vi "3_Axis_magmeter_MAIN.vi"() -> ()   [LabVIEW 2013]
doc: "Программа для обработки и визуализации трех компонент магнитного поля прибора, разработаного инженерами НЭОиКН ЛФВЭ ОИЯИ 2014"
uses:
  Magmeter.ctl
  <vilib>/Instr/_visa.llb/VISA Configure Serial Port (Instr).vi
panel:
  out "Dx Sum":u64
  in  "Порт":refnum<visa-resource-name>="COM4"
  out "Соединение":bool
  out "Err msg":string=" INSTRUCTIONS:\r\rNormal Use:  When using subVIs that incorporate the error in/error out (or error I/O) structure, place this handler where you want to inform the user of an error, typically at the end of the I/O data path, as the last action of the program.  If the error in error? is ERROR, the handler creates a message describing the error and its source.  If the type of dialog = 1 (default), the message is displayed to the user, who can only acknowedge it.  If the type = 2, the user can acknowledge the message or abort execution; aborting a program with active I/O is not recommended.  If the type = 0, no message is displayed; this is used to process the error programmatically, and the error out cluster elements are wired to individual terminals for that reason.  \r\rOther Use:\n\r\nlocal testing.  To test the error code of a subVI or function that does not have the error I/O structure, you can wire its error code and a source string to the local error code and error source inputs.  If error in error? indicates no error and error code is not equal to 0, the local code and source are substituted for the error in values, and error? is set TRUE (ERROR)."
  in  "Бод.":u32=9600
  out "i":i32
  in  "number of data sample":u64
  in  "Автосохранение":bool
  in  "Интервал \n\n[сек.]":u32=10 min=1 max=30000 step=1
  in  "Маркеры":bool
  out "Table num index":u32
  in  "Удалить измерение":bool
  in  "RXd number":u64
  in  "Dz, мм":u64=5 min=1
  in  "зафиксировать измерение":bool
  in  "Измерений\n \nна графике":u16=100
  in  "Очистить историю":bool
  in  "H макс":dbl=8.0 format="%#.1f"
  in  "H мин":dbl=-8.0 format="%#.1f"
  in  "Уст. ноль":bool
  in  "Сохранен!":bool
  in  "Plot.Visible Z":bool
  out "By":dbl format="%.3f"
  out "Bz":dbl format="%.3f"
  in  "Plot.Visible X":bool
  out "Bx":dbl format="%.3f"
  in  "Plot.Visible Y":bool
  in  "Графики толще":bool=TRUE
  in  "Стоп":bool
  out "Магнитные измерения":T1(graph)
  in  "Measurment Fl":bool
  out "Сохраненные измерения":string[][](table)
  out "Путь к файлу":path
  # "Гаусс"
  # "Результаты\nизмерений"
  # "ГС"
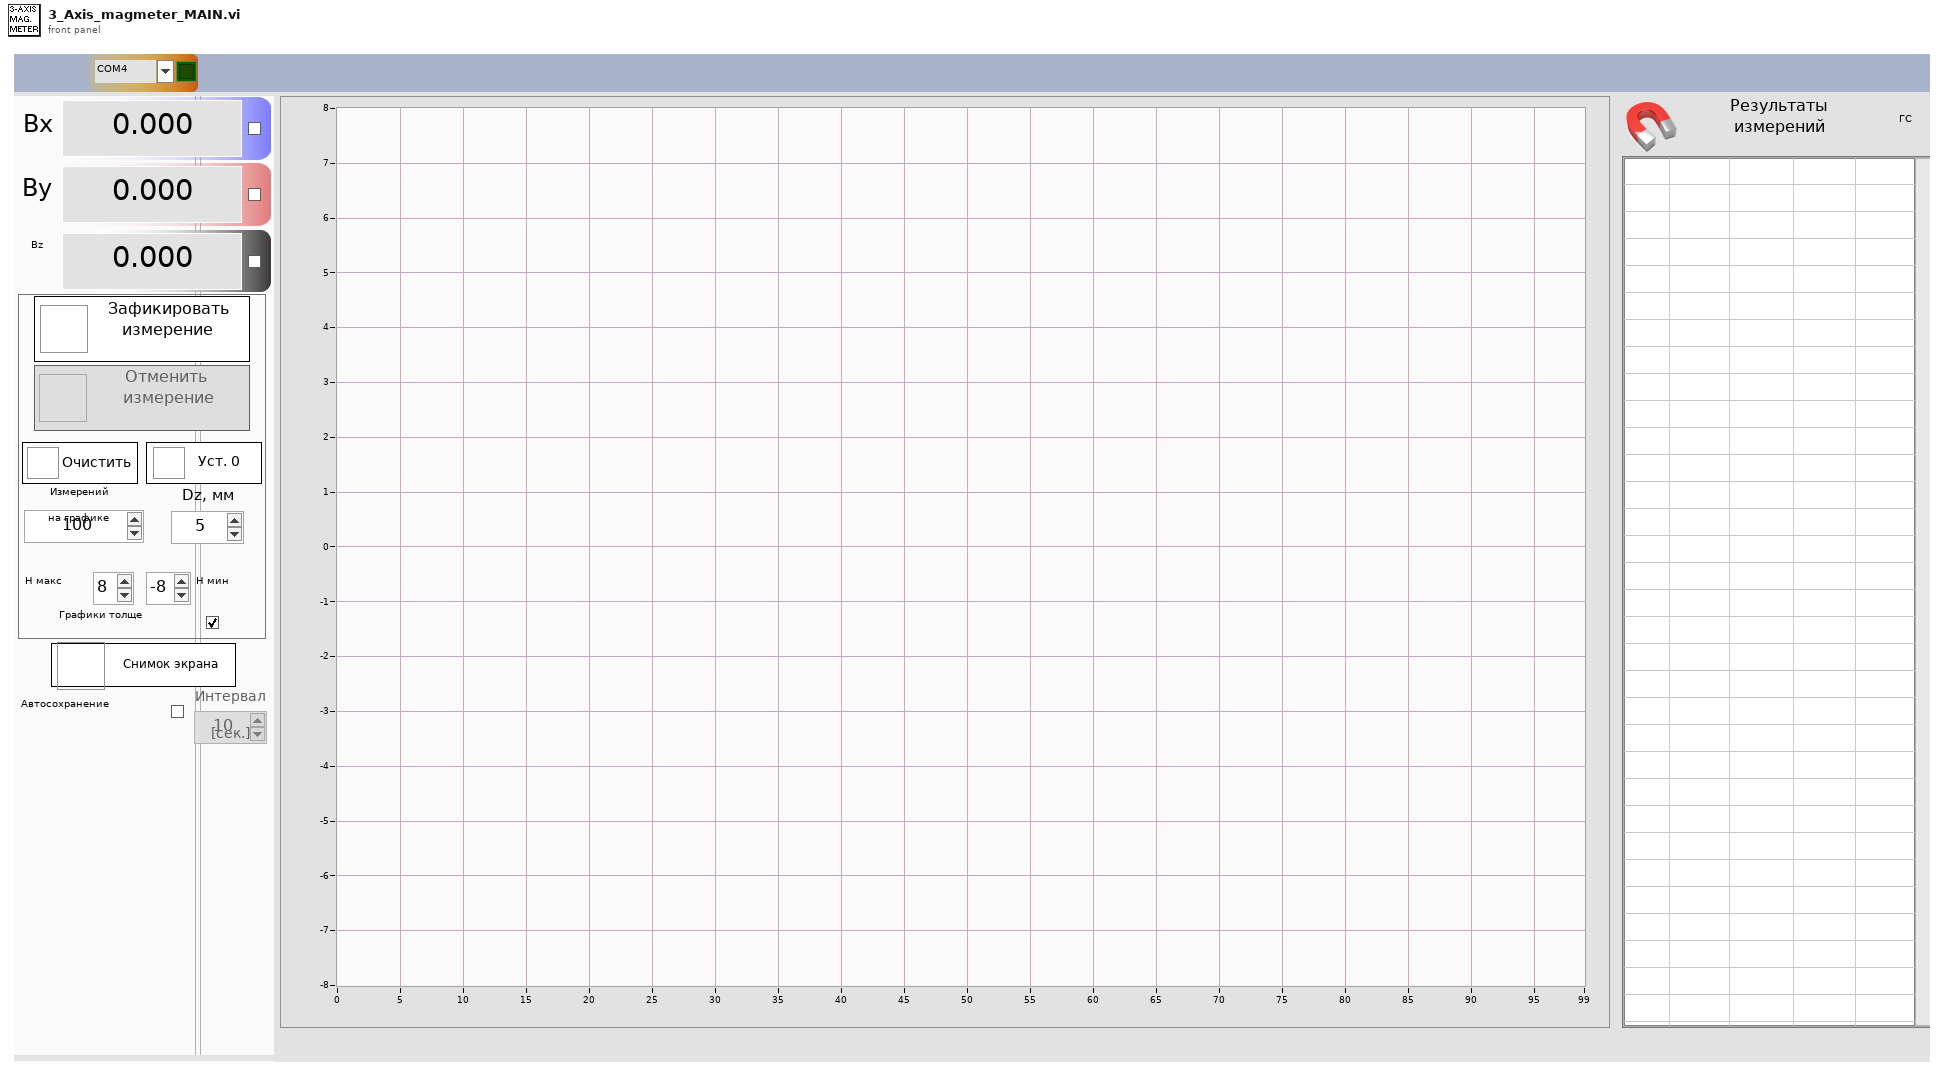
[diagram p1: front panel]
types:
  T1 = cluster{"X":dbl, "Y":dbl, "Z":dbl, "Active Plot":dbl}[]
  T2 = typedef "Magmeter.ctl" = enum16{"Initialize", "Read port", "Write port", "Stop"}
  T3 = cluster{"Value":dbl, "Value":dbl, "Value":dbl, "Active Plot":dbl}
  T4 = cluster{"Value":dbl, "Value":dbl, "Value":dbl, "X":dbl}
  T5 = cluster{"Value":dbl, "Value":dbl, "Value":dbl, "X":dbl}[]
  T6 = typedef "imagedata.ctl" = cluster{"image type":i32, "image depth":i32, "image":u8[], "mask":u8[], "colors":u32[], "Rectangle":cluster{"left":i16, "top":i16, "right":i16, "bottom":i16}}
  T7 = cluster{"read buffer":string, "serial out":refnum<visa-resource-name>, "error out":errorcluster, "occurrence":refnum<k4>}
  T8 = cluster{"out string":string, "Visa name out":refnum<visa-resource-name>, "error out":errorcluster, "occurrence":refnum<k4>}
  T9 = cluster{"Visa name out":refnum<visa-resource-name>, "error out":errorcluster, "status":bool, "occurrence":refnum<k4>}
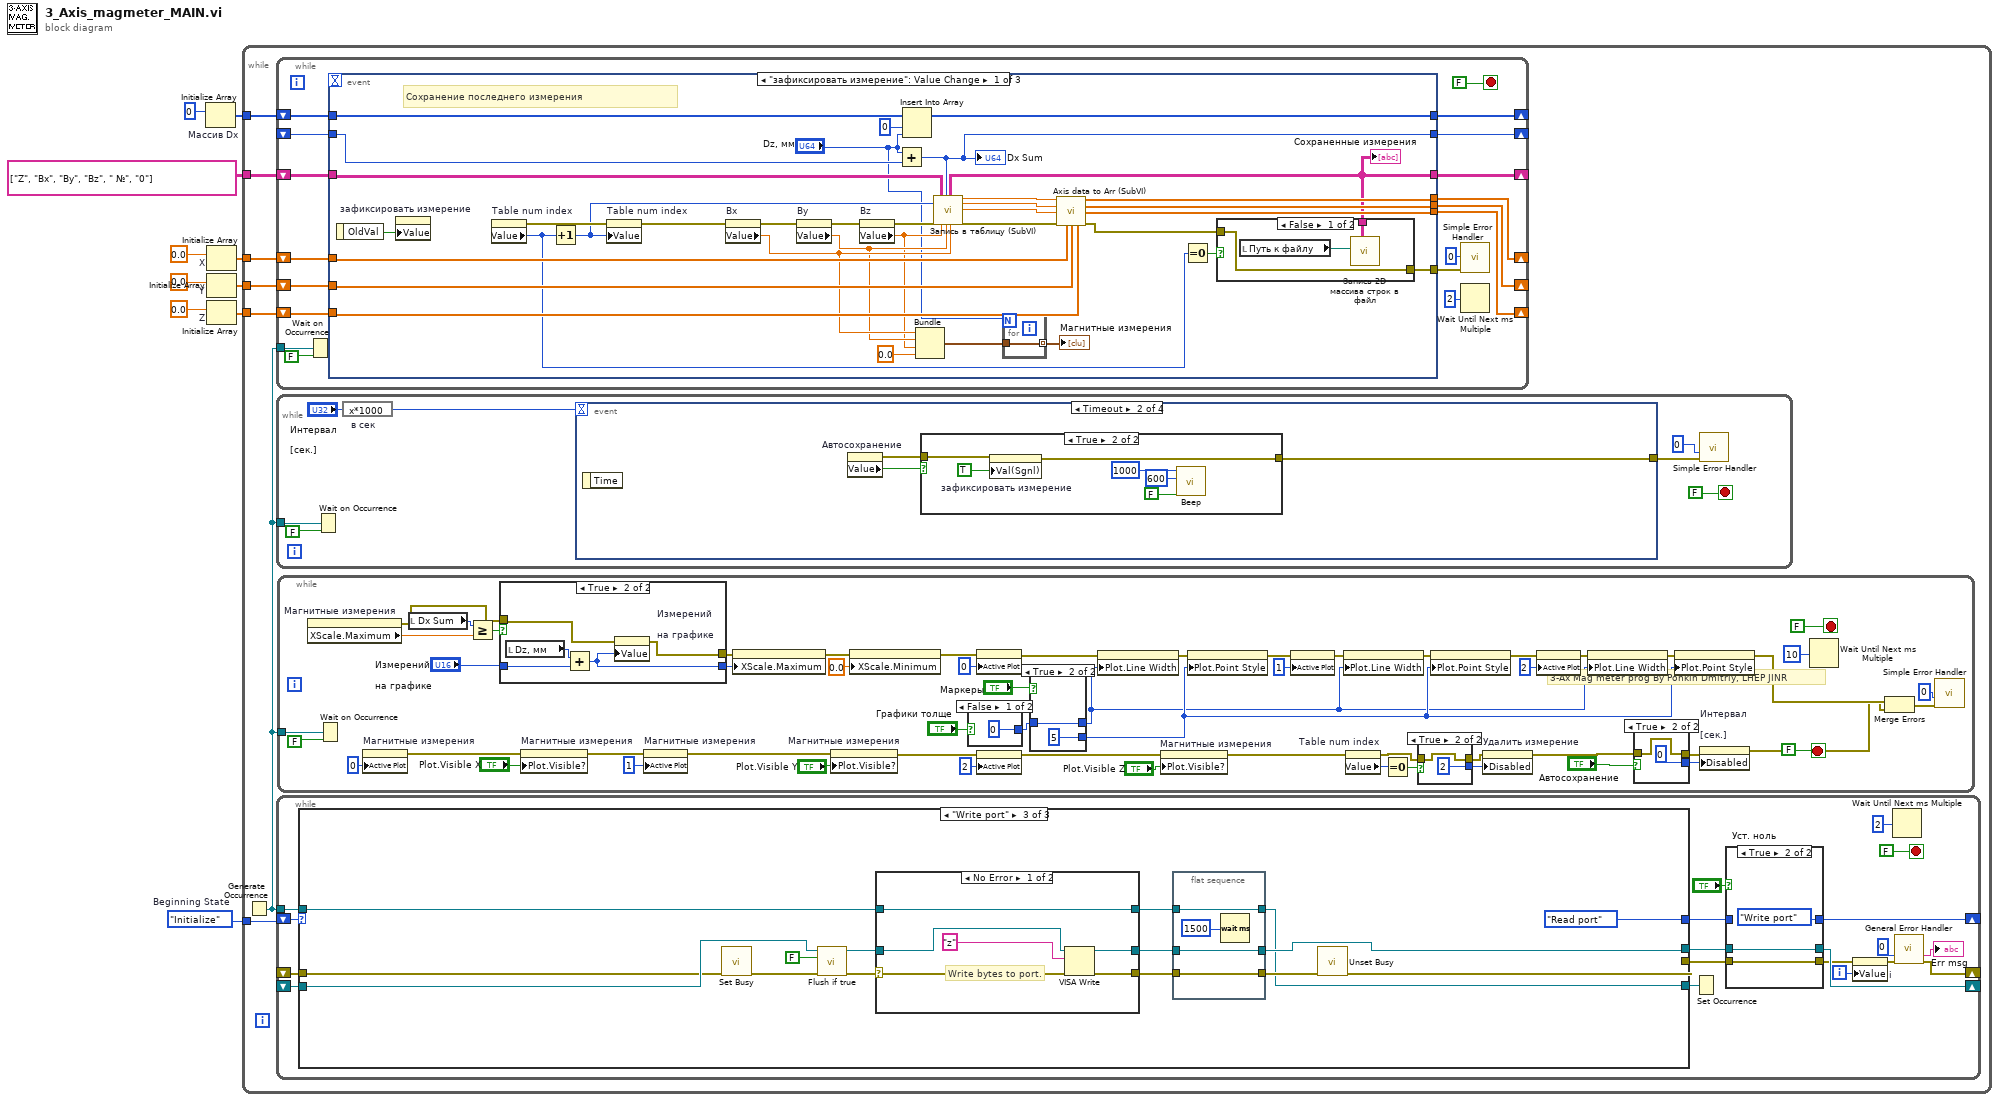
[diagram p0: block diagram]
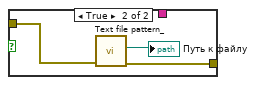
[diagram p2: hidden frame]
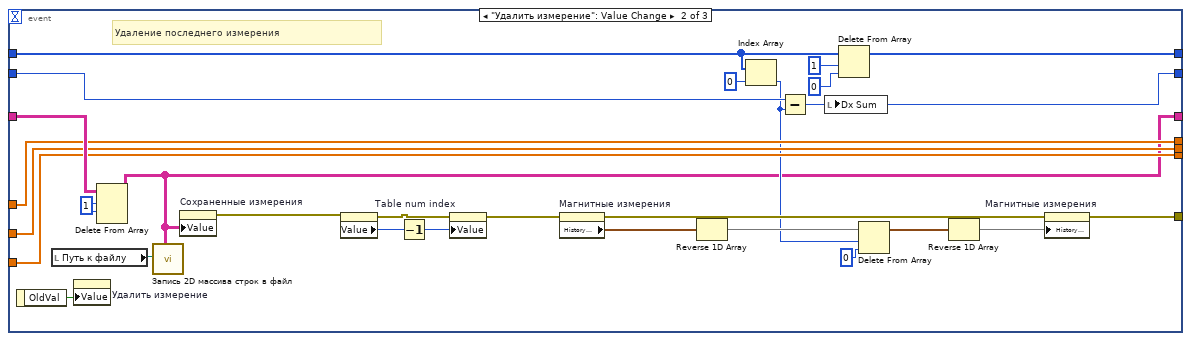
[diagram p3: hidden frame]
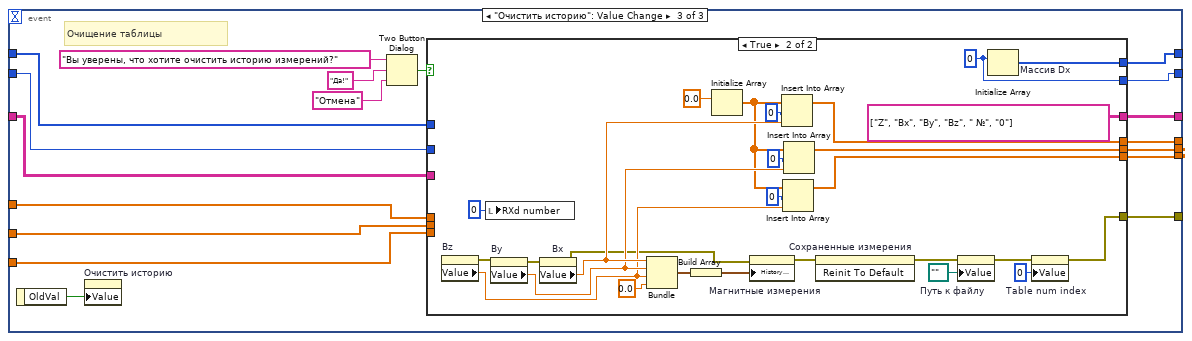
[diagram p4: hidden frame]
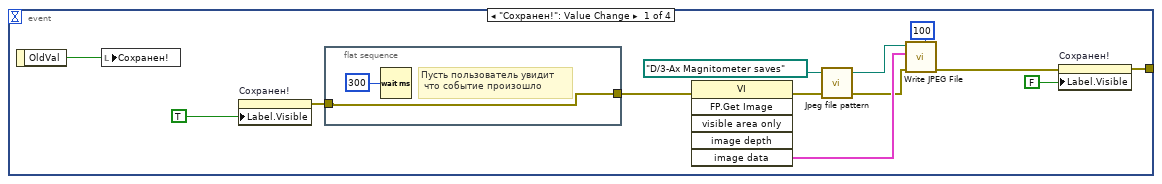
[diagram p6: hidden frame]
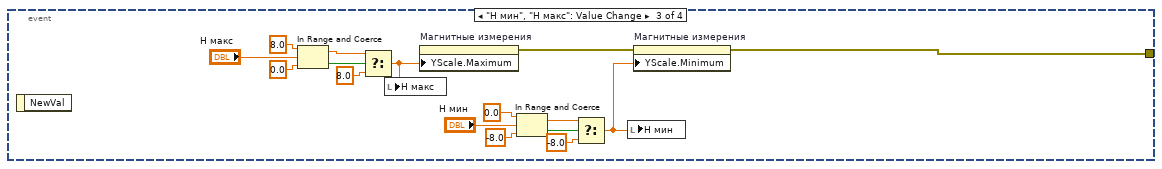
[diagram p8: hidden frame]
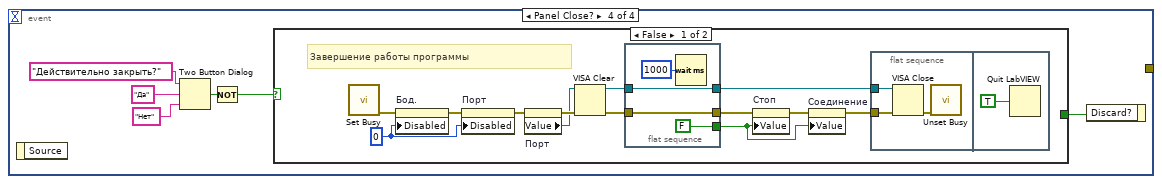
[diagram p9: hidden frame]
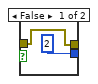
[diagram p11: hidden frame]
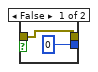
[diagram p12: hidden frame]
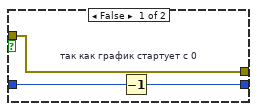
[diagram p13: hidden frame]
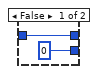
[diagram p14: hidden frame]
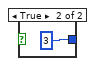
[diagram p15: hidden frame]
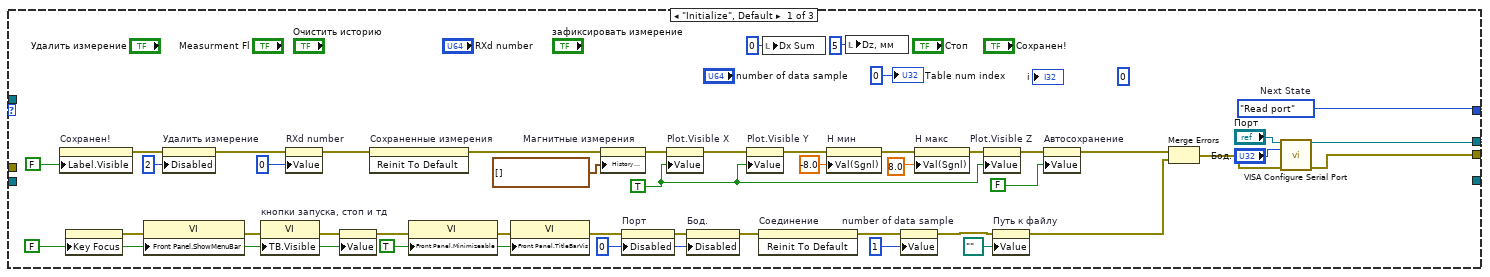
[diagram p17: hidden frame]
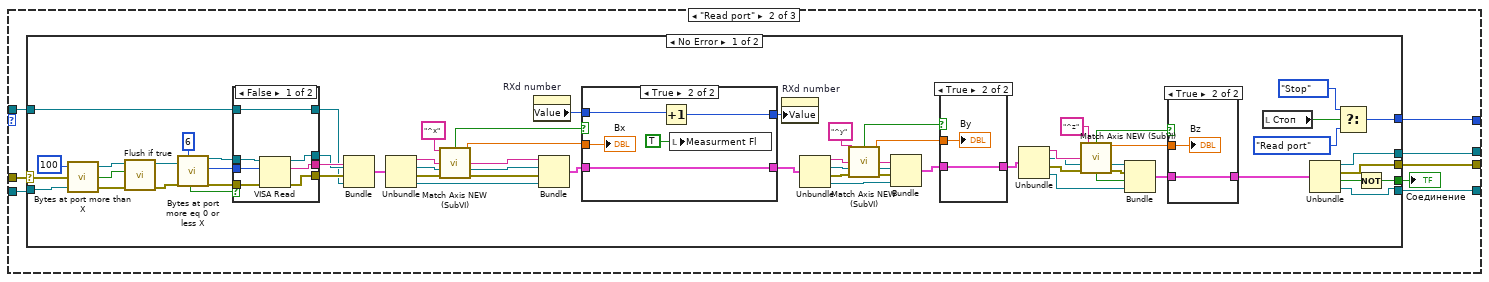
[diagram p18: hidden frame]
diagram:
  w10 = Magmeter."Initialize"  # Beginning State
  n1 = Initialize Array "Массив Dx"(u64 0 ("element")) -> (w1:u64[])  [unwired: 1 out]
  n2 = Initialize Array "X"(0.0 ("element")) -> (w7:dbl[])  [unwired: 1 out]
  n3 = Initialize Array "Y"(0.0 ("element")) -> (w4:dbl[])  [unwired: 1 out]
  n4 = Initialize Array "Z"(0.0 ("element")) -> (w3:dbl[])  [unwired: 1 out]
  n5 = while {
    tunnel: w10 -> [w18]
    tunnel: string[][] [["Z", "Bx", "By", "Bz", " №", "0"]] ("Сохраненные измерения") -> [w16]
    tunnel: w7 -> [w15]
    tunnel: w4 -> [w13]
    tunnel: w3 -> [w12]
    tunnel: w1 -> [w11]
    stop <- FALSE stop-if-true
    # "3-Ax Mag meter prog By Ponkin Dmitriy, LHEP JINR"
    n6 = Generate Occurrence() -> (w14:refnum<k4>)
    n7 = while {
      shift-right: [w36] -> _
      shift-left: w16 -> [w35]
      shift-right: [w33] -> _
      shift-left: w15 -> [w34]
      tunnel: w14 -> [w30]
      shift-right: [w24] -> _
      shift-left: w12 -> [w26]
      shift-right: [w25] -> _
      shift-left: w13 -> [w27]
      shift-right: [w23] -> _
      shift-left: w11 -> [w22]
      shift-right: [w21] -> _
      shift-left: _ -> [w20]
      stop <- FALSE stop-if-true
      n8 = Wait on Occurrence(1:FALSE ("ignore previous (T)"), 2:w30) -> ()  [unwired: 1 in, 1 out]
      n9 = event shown="[0] \"зафиксировать измерение\": Value Change" {
        selector: _ -> [_ _ _]
        dyn-events: _ -> [_ _ _]
        timeout: _ -> [_ _ _]
        tunnel: w35 -> [w55 w104 w122]
        tunnel: [w37 w90 w123] -> w32
        tunnel: [w40 w80 w124] -> w36
        tunnel: w34 -> [w62 w102 w116]
        tunnel: [w59 w102 w117] -> w33
        tunnel: w27 -> [w61 w100 w115]
        tunnel: w26 -> [w60 w99 w114]
        tunnel: [w58 w99 w112] -> w24
        tunnel: [w57 w100 w113] -> w25
        tunnel: [w50 w87 w111] -> w23
        tunnel: w22 -> [w53 w82 w108]
        tunnel: [w52 w83 w110] -> w21
        tunnel: w20 -> [w51 w85 w109]
        event "зафиксировать измерение": Value Change {
          # "Сохранение последнего измерения"
          n10 = event-data() -> ("OldVal"=w47:bool)  [unwired: 1 out]
          n11 = property on="зафиксировать измерение" class="Bool (strict)"("Value"=w47) -> ()  [unwired: 2 in, 2 out]
          n12 = property on="Table num index" class="DigNum (strict)"() -> (error out=w71:errorcluster, "Value"=w39:u32)  [unwired: 2 in, 1 out]
          n13 = Increment(x=w39) -> (x+1=w56:u32)
          n14 = property on="Table num index" class="DigNum (strict)"(error in=w71, "Value"=w56) -> (error out=w68:errorcluster)  [unwired: 1 in, 1 out]
          n15 = property on="Bx" class="DigNum (strict)"(error in=w68) -> (error out=w70:errorcluster, "Value"=w46:dbl)  [unwired: 1 in, 1 out]
          n16 = property on="By" class="DigNum (strict)"(error in=w70) -> (error out=w69:errorcluster, "Value"=w45:dbl)  [unwired: 1 in, 1 out]
          n17 = property on="Bz" class="DigNum (strict)"(error in=w69) -> (error out=w67:errorcluster, "Value"=w44:dbl)  [unwired: 1 in, 1 out]
          n18 = Add(x="Dz, мм", y=w51) -> (x+y=w52:u64)
          "Dx Sum" <- w52
          n19 = Insert Into Array "Insert Into Array"(array=w53, index=0, new element="Dz, мм") -> (w50:u64[])
          n20 = Bundle("Value"=w46, "Value"=w45, "Value"=w44, "Active Plot"=0.0) -> (w49:T3)  [unwired: 1 out]
          n21 = call "Запись в таблицу (SubVI).vi"("data num"=w56, "error in"=w67, "String Arr in"=w55, "Z axis data"=w44, "Шаг измерений"=w52, "Y axis data"=w45, "X axis data"=w46) -> ("String Arr out"=w40:string[][], "X axis data out"=w65:dbl, "Y axis data out"=w64:dbl, "Z axis data out"=w63:dbl, "error out"=w66:errorcluster)  [unwired: 5 in, 3 out]
          "Сохраненные измерения" <- w40
          n22 = for {
            N: "Dz, мм" -> [_]
            tunnel: [w78] -> w42 mode=indexing
            tunnel: w49 -> [w78]
          }
          "Магнитные измерения" <- w42
          n23 = call "Axis data to Arr (SubVI).vi"("new X element"=w65, "new Y element"=w64, "new Z element"=w63, "error in"=w66, "X Arr in"=w62, "Y Arr in"=w61, "Z Arr in"=w60) -> ("X Arr Out"=w59:dbl[], "Y Arr Out"=w57:dbl[], "Z Arr Out"=w58:dbl[], "error out"=w38:errorcluster)  [unwired: 5 out]
          n24 = Equal To 0?(x=w39) -> (x = 0?=w41:bool)
          n25 = case shown="False" w41 {
            tunnel: w40 -> [w74 _]
            tunnel: w38 -> [w72 w76]
            tunnel: [w72 w75] -> w37
            frame False {
              n26 = local read "Путь к файлу"() -> (w73:path)
              n27 = call "Запись 2D массива строк в файл.vi"("путь к файлу"=w73, "2-D массив строк для записи"=w74) -> ()  [unwired: 2 in, 16 out]
            }
            frame True {
              n28 = call "Text file pattern_.vi"("error in"=w76) -> ("error out"=w75:errorcluster, "путь к файлу"=→"Путь к файлу":path)  [unwired: 9 out]
            }
          }
        }
        event "Удалить измерение": Value Change {
          w103 = 1 ("length")
          # "Удаление последнего измерения"
          n29 = event-data() -> ("OldVal"=w81:bool)  [unwired: 1 out]
          n30 = local read "Путь к файлу"() -> (w79:path)
          n31 = property on="Удалить измерение" class="Bool (strict)"("Value"=w81) -> ()  [unwired: 2 in, 2 out]
          n32 = Delete From Array "Delete From Array"(array=w104, length=w103, index (row)=w103) -> (array with subset deleted=w80:string[][])  [unwired: 1 in, 1 out]
          n33 = call "Запись 2D массива строк в файл.vi"("путь к файлу"=w79, "2-D массив строк для записи"=w80) -> ()  [unwired: 2 in, 16 out]
          n34 = property on="Сохраненные измерения" class="Tbl (strict)"("Value"=w80) -> (error out=w91:errorcluster)  [unwired: 2 in, 1 out]
          n35 = property on="Table num index" class="DigNum (strict)"(error in=w91) -> (error out=w101:errorcluster, "Value"=w106:u32)  [unwired: 1 in, 1 out]
          n36 = Decrement(x=w106) -> (x-1=w105:u32)
          n37 = property on="Table num index" class="DigNum (strict)"(error in=w101, "Value"=w105) -> (error out=w92:errorcluster)  [unwired: 1 in, 1 out]
          n38 = property on="Магнитные измерения" class="WFChart (strict)"(error in=w92) -> (error out=w93:errorcluster, "History Data"=w97:T1)  [unwired: 1 in, 1 out]
          n39 = Reverse 1D Array(array=w97) -> (reversed array=w96:T1)
          n40 = Index Array "Index Array"(array=w82, index=0) -> (element=w84:u64)
          n41 = Subtract(x=w85, y=w84) -> (x-y=w83:u64)
          n42 = local write "Dx Sum"(w83) -> ()
          n43 = Delete From Array "Delete From Array"(array=w82, length=1, index=0 ("length")) -> (array with subset deleted=w87:u64[])  [unwired: 1 out]
          n44 = Delete From Array "Delete From Array"(array=w96, length=w84, index=0 ("length")) -> (array with subset deleted=w94:T1)  [unwired: 1 out]
          n45 = Reverse 1D Array(array=w94) -> (reversed array=w95:T1)
          n46 = property on="Магнитные измерения" class="WFChart (strict)"(error in=w93, "History Data"=w95) -> (error out=w90:errorcluster)  [unwired: 1 in, 1 out]
        }
        event "Очистить историю": Value Change {
          # "Очищение таблицы"
          n47 = event-data() -> ("OldVal"=w107:bool)  [unwired: 1 out]
          n48 = property on="Очистить историю" class="Bool (strict)"("Value"=w107) -> ()  [unwired: 2 in, 2 out]
          n49 = Two Button Dialog(message="Вы уверены, что хотите очистить историю измерений?", 1:"Отмена" ("T button name (\"OK\")"), 2:"Да!" ("T button name (\"OK\")")) -> (T button?=w118:bool)
          n50 = case shown="True" w118 {
            tunnel: [w130 string[][] [["Z", "Bx", "By", "Bz", " №", "0"]] ("Сохраненные измерения")] -> w124
            tunnel: [_ w137] -> w123
            tunnel: w122 -> [w130 _]
            tunnel: [w129 w150] -> w117
            tunnel: w116 -> [w129 _]
            tunnel: w115 -> [w128 _]
            tunnel: w114 -> [w127 _]
            tunnel: [w128 w145] -> w113
            tunnel: [w127 w143] -> w112
            tunnel: w108 -> [w126 _]
            tunnel: [w126 w136] -> w111
            tunnel: [w125 w135] -> w110
            tunnel: w109 -> [w125 _]
            frame False {
            }
            frame True {
              w135 = u64 0 ("element")
              n51 = property on="Bz" class="DigNum (strict)"() -> (error out=w140:errorcluster, "Value"=w142:dbl)  [unwired: 2 in, 1 out]
              n52 = local write "RXd number"(u64 0 ("RXd number")) -> ()
              n53 = property on="By" class="DigNum (strict)"(error in=w140) -> (error out=w139:errorcluster, "Value"=w146:dbl)  [unwired: 1 in, 1 out]
              n54 = property on="Bx" class="DigNum (strict)"(error in=w139) -> (error out=w138:errorcluster, "Value"=w147:dbl)  [unwired: 1 in, 1 out]
              n55 = Bundle("Value"=w147, "Value"=w146, "Value"=w142, "X"=0.0) -> (w153:T4)  [unwired: 1 out]
              n56 = Build Array(w153) -> (w148:T5)
              n57 = Initialize Array(0.0 ("element")) -> (w141:dbl[])  [unwired: 1 out]
              n58 = property on="Магнитные измерения" class="WFChart (strict)"(error in=w138, "History Data"=w148) -> (error out=w155:errorcluster)  [unwired: 1 in, 1 out]
              n59 = Insert Into Array(array=w141, index=0, new element=w147) -> (w150:dbl[])
              n60 = Insert Into Array(array=w141, index=0, new element=w142) -> (w143:dbl[])
              n61 = Insert Into Array(array=w141, index=0, new element=w146) -> (w145:dbl[])
              n62 = invoke on="Сохраненные измерения" class="Tbl (strict)" method="Reinit To Default"(error in=w155) -> (error out=w132:errorcluster)  [unwired: 2 in, 2 out]
              n63 = property on="Путь к файлу" class="Path"(error in=w132, "Value"=path "" ("Путь к файлу")) -> (error out=w131:errorcluster)  [unwired: 1 in, 1 out]
              n64 = Initialize Array "Массив Dx"(w135) -> (w136:u64[])  [unwired: 1 out]
              n65 = property on="Table num index" class="DigNum (strict)"(error in=w131, "Value"=u32 0 ("Table num index")) -> (error out=w137:errorcluster)  [unwired: 1 in, 1 out]
            }
          }
        }
      }
      n66 = call <vilib>:"Simple Error Handler.vi"("type of dialog (OK msg:1)"=u32 0 ("Table num index"), "error in (no error)"=w32) -> ()  [unwired: 8 out]
      n67 = Wait Until Next ms Multiple(millisecond multiple=u32 2) -> ()  [unwired: 1 out]
    }
    n68 = while {
      tunnel: w14 -> [w161]
      stop <- FALSE stop-if-true
      n69 = Wait on Occurrence(1:FALSE ("ignore previous (T)"), 2:w161) -> ()  [unwired: 1 in, 1 out]
      n70 = expression code="x*1000" "в сек"("Интервал \n\n[сек.]") -> (w158:u32)
      n71 = event shown="[1] Timeout" {
        selector: _ -> [_ _ _ _]
        dyn-events: _ -> [_ _ _ _]
        timeout: w158 -> [_ _ _ _]
        tunnel: [w171 w182 w190 _] -> w163
        event "Сохранен!": Value Change {
          n72 = event-data() -> ("OldVal"=w172:bool)  [unwired: 1 out]
          n73 = local write "Сохранен!"(w172) -> ()
          n74 = property on="Сохранен!" class="Bool (strict)"("Label.Visible"=TRUE) -> (error out=w166:errorcluster)  [unwired: 2 in, 1 out]
          n75 = flat-sequence {
            tunnel: [w178] -> w167
            tunnel: w166 -> [w178]
            frame #0 {
              # "Пусть пользователь увидит\n что событие произошло"
              n76 = Wait (ms)(milliseconds to wait=u32 300) -> ()  [unwired: 1 out]
            }
          }
          n77 = invoke class="VI" method="FP.Get Image"(error in=w167) -> (error out=w175:errorcluster, "image data"=w176:T6)  [unwired: 5 in, 4 out]
          n78 = call "Jpeg file pattern.vi"("path"=path "D:/3-Ax Magnitometer saves" ("path (use dialog)"), "error in"=w175) -> ("path to JPG file"=w174:path, "error out"=w173:errorcluster)  [unwired: 6 out]
          n79 = call <vilib>:"Write JPEG File.vi"("quality (80)"=100, "error in (no error)"=w173, "image data"=w176, "path to JPEG file"=w174) -> ("error out"=w170:errorcluster)  [unwired: 7 out]
          n80 = property on="Сохранен!" class="Bool (strict)"(error in=w170, "Label.Visible"=FALSE) -> (error out=w171:errorcluster)  [unwired: 1 in, 1 out]
        }
        event Timeout {
          n81 = event-data() -> ()  [unwired: 2 out]
          n82 = property on="Автосохранение" class="Bool (strict)"() -> (error out=w180:errorcluster, "Value"=w181:bool)  [unwired: 2 in, 1 out]
          n83 = case shown="True" w181 {
            tunnel: [w183 w188] -> w182
            tunnel: w180 -> [w183 w187]
            frame False {
            }
            frame True {
              n84 = property on="зафиксировать измерение" class="Bool (strict)"(error in=w187, "Val(Sgnl)"=TRUE ("Value (Signaling)")) -> (error out=w188:errorcluster)  [unwired: 1 in, 1 out]
              n85 = call <vilib>:"Beep.vi"("use system alert? (T)"=FALSE, "duration (msec)"=u32 600, "frequency (Hz)"=u32 1000 ("duration (msec)")) -> ()  [unwired: 9 out]
            }
          }
        }
        event "H мин", "H макс": Value Change {
          n86 = event-data() -> ()  [unwired: 2 out]
          n87 = In Range and Coerce(upper limit=8.0, x="H макс", lower limit=0.0) -> (coerced(x)=w201:dbl, In Range?=w203:bool)
          n88 = Select(t=w201, s=w203, f=8.0) -> (s? t:f=w193:dbl)
          n89 = local write "H макс"(w193) -> ()
          n90 = property on="Магнитные измерения" class="WFChart (strict)"("YScale.Maximum"=w193) -> (error out=w191:errorcluster)  [unwired: 2 in, 1 out]
          n91 = In Range and Coerce(upper limit=0.0, x="H мин", lower limit=-8.0) -> (coerced(x)=w199:dbl, In Range?=w197:bool)
          n92 = Select(t=w199, s=w197, f=-8.0) -> (s? t:f=w192:dbl)
          n93 = local write "H мин"(w192) -> ()
          n94 = property on="Магнитные измерения" class="WFChart (strict)"(error in=w191, "YScale.Minimum"=w192) -> (error out=w190:errorcluster)  [unwired: 1 in, 1 out]
        }
        event Panel Close? {
          n95 = event-data() -> ()  [unwired: 2 out]
          n96 = Two Button Dialog(message="Действительно закрыть?", 1:"Нет", 2:"Да") -> (T button?=w208:bool)
          n97 = Not(x=w208) -> (.not. x?=w207:bool)
          n98 = case shown="False" w207 {
            selector: w207 -> [_ w233]
            tunnel: [_ w233] -> w206
            frame False {
              w221 = u8 0 ("Disabled")
              # "Завершение работы программы"
              n99 = call <vilib>:"Set Busy.vi"() -> ("error out"=w213:errorcluster)  [unwired: 4 in, 7 out]
              n100 = property on="Бод." class="DigNum (strict)"(error in=w213, "Disabled"=w221) -> (error out=w224:errorcluster)  [unwired: 1 in, 1 out]
              n101 = property on="Порт" class="VISAName"(error in=w224, "Disabled"=w221) -> (error out=w212:errorcluster)  [unwired: 1 in, 1 out]
              n102 = property on="Порт" class="VISAName"(error in=w212) -> (error out=w215:errorcluster, "Value"=w214:refnum<visa-resource-name>)  [unwired: 1 in, 1 out]
              n103 = VISA Clear(VISA resource name=w214, error in (no error)=w215) -> (VISA resource name out=w223:refnum<visa-resource-name>, error out=w222:errorcluster)
              n104 = flat-sequence {
                tunnel: w223 -> [w227]
                tunnel: [w227] -> w219
                tunnel: [w226] -> w217
                tunnel: w222 -> [w226]
                tunnel: [FALSE ("Visible")] -> w216
                frame #0 {
                  n105 = Wait (ms)(milliseconds to wait=u32 1000) -> ()  [unwired: 1 out]
                }
              }
              n106 = property on="Стоп" class="Bool (strict)"(error in=w217, "Value"=w216) -> (error out=w218:errorcluster)  [unwired: 1 in, 1 out]
              n107 = property on="Соединение" class="Bool (strict)"(error in=w218, "Value"=w216) -> (error out=w220:errorcluster)  [unwired: 1 in, 1 out]
              n108 = flat-sequence {
                tunnel: w220 -> [w231]
                tunnel: w219 -> [w230]
                frame #0 {
                  n109 = VISA Close(VISA resource name=w230, error in (no error)=w231) -> (error out=w229:errorcluster)
                  n110 = call <vilib>:"Unset Busy.vi"("error in (no error)"=w229) -> ()  [unwired: 1 in, 10 out]
                }
                frame #1 {
                  n111 = Quit LabVIEW(quit? (T)=TRUE ("stop? (T)")) -> ()
                }
              }
            }
            frame True {
            }
          }
          n112 = event-data("Discard?"=w206) -> ()  [unwired: 1 in, 1 out]
        }
      }
      n113 = call <vilib>:"Simple Error Handler.vi"("type of dialog (OK msg:1)"=u32 0 ("Table num index"), "error in (no error)"=w163) -> ()  [unwired: 8 out]
    }
    n114 = while "While sa" {
      shift-right: [w320] -> _
      shift-left: w18 -> [w329]
      shift-right: [w312] -> _
      shift-left: _ -> [w326]
      tunnel: w14 -> [w323]
      shift-right: [w318] -> _
      shift-left: _ -> [w322]
      i -> [w325]
      stop <- FALSE stop-if-true
      n115 = case shown="\"Write port\"" w329 {
        tunnel: [w374 w381 Magmeter."Read port" ("Beginning State")] -> w321
        tunnel: w326 -> [_ w384 w493]
        tunnel: w323 -> [_ w386 w497]
        tunnel: w322 -> [_ w385 w495]
        tunnel: [w359 w380 w487] -> w317
        tunnel: [w358 w383 w492] -> w315
        tunnel: [_ w382 w486] -> w316
        frame "Initialize", Default {
          (unwired) u64 0 ("ост. вр")
          w374 = Magmeter."Read port"  # Next State
          w340 = TRUE ("Plot.Visible X")
          w371 = TRUE ("Front Panel Window:Minimizable")
          w368 = FALSE ("Front Panel Window:Resizable")
          w369 = u8 0 ("Disabled")
          n116 = property on="Сохранен!" class="Bool (strict)"("Label.Visible"=FALSE) -> (error out=w352:errorcluster)  [unwired: 2 in, 1 out]
          n117 = property on="Стоп" class="Bool (strict)"("Key Focus"=w368) -> (error out=w373:errorcluster)  [unwired: 2 in, 1 out]
          n118 = property class="VI"(error in=w373, "Front Panel.ShowMenuBar"=w368) -> (error out=w372:errorcluster)  [unwired: 1 in, 1 out]
          n119 = property on="Удалить измерение" class="Bool (strict)"(error in=w352, "Disabled"=u8 2) -> (error out=w354:errorcluster)  [unwired: 1 in, 1 out]
          n120 = property on="кнопки запуска, стоп и тд" class="VI"(error in=w372, "TB.Visible"=w368) -> (error out=w367:errorcluster)  [unwired: 1 in, 1 out]
          n121 = property on="RXd number" class="DigNum (strict)"(error in=w354, "Value"=u64 0 ("RXd number")) -> (error out=w355:errorcluster)  [unwired: 1 in, 1 out]
          n122 = property on="Стоп" class="Bool (strict)"(error in=w367, "Value"=w368) -> (error out=w364:errorcluster)  [unwired: 1 in, 1 out]
          n123 = invoke on="Сохраненные измерения" class="Tbl (strict)" method="Reinit To Default"(error in=w355) -> (error out=w356:errorcluster)  [unwired: 2 in, 2 out]
          n124 = property class="VI"(error in=w364, "Front Panel.Minimizeable"=w371) -> (error out=w370:errorcluster)  [unwired: 1 in, 1 out]
          n125 = property class="VI"(error in=w370, "Front Panel.TitleBarVis"=w371) -> (error out=w365:errorcluster)  [unwired: 1 in, 1 out]
          n126 = property on="Магнитные измерения" class="WFChart (strict)"(error in=w356, "History Data"=T1 []) -> (error out=w360:errorcluster)  [unwired: 1 in, 1 out]
          n127 = property on="Порт" class="VISAName"(error in=w365, "Disabled"=w369) -> (error out=w366:errorcluster)  [unwired: 1 in, 1 out]
          n128 = property on="Plot.Visible X" class="Bool (strict)"(error in=w360, "Value"=w340) -> (error out=w362:errorcluster)  [unwired: 1 in, 1 out]
          n129 = property on="Бод." class="DigNum (strict)"(error in=w366, "Disabled"=w369) -> (error out=w375:errorcluster)  [unwired: 1 in, 1 out]
          n130 = property on="Plot.Visible Y" class="Bool (strict)"(error in=w362, "Value"=w340) -> (error out=w349:errorcluster)  [unwired: 1 in, 1 out]
          n131 = invoke on="Соединение" class="Bool (strict)" method="Reinit To Default"(error in=w375) -> (error out=w378:errorcluster)  [unwired: 2 in, 2 out]
          n132 = local write "Dx Sum"(u64 0 ("Dx Sum")) -> ()
          n133 = property on="H мин" class="DigNum (strict)"(error in=w349, "Val(Sgnl)"=-8.0 ("Value (Signaling)")) -> (error out=w347:errorcluster)  [unwired: 1 in, 1 out]
          n134 = local write "Dz, мм"(u64 5 ("Dz, мм")) -> ()
          n135 = property on="number of data sample" class="DigNum (strict)"(error in=w378, "Value"=u64 1 ("number of data sample")) -> (error out=w341:errorcluster)  [unwired: 1 in, 1 out]
          n136 = property on="H макс" class="DigNum (strict)"(error in=w347, "Val(Sgnl)"=8.0 ("Value (Signaling)")) -> (error out=w346:errorcluster)  [unwired: 1 in, 1 out]
          n137 = property on="Plot.Visible Z" class="Bool (strict)"(error in=w346, "Value"=w340) -> (error out=w339:errorcluster)  [unwired: 1 in, 1 out]
          n138 = property on="Путь к файлу" class="Path"(error in=w341, "Value"=path "" ("Путь к файлу")) -> (error out=w337:errorcluster)  [unwired: 1 in, 1 out]
          n139 = property on="Автосохранение" class="Bool (strict)"(error in=w339, "Value"=FALSE ("Plot.Visible X")) -> (error out=w338:errorcluster)  [unwired: 1 in, 1 out]
          n140 = Merge Errors(w338, w337) -> (w343:errorcluster)
          n141 = call-poly "VISA Configure Serial Port"("VISA resource name"="Порт", "baud rate (9600)"="Бод.", "error in (no error)"=w343) -> ("VISA resource name out"=w359:refnum<visa-resource-name>, "error out"=w358:errorcluster)  [unwired: 3 in, 8 out]
          "Table num index" <- u32 0 ("Table num index")
        }
        frame "Read port" {
          n142 = case shown="No Error" w384 {
            selector: w384 -> [w432 w484]
            tunnel: [w451 w480] -> w381
            tunnel: [w403 FALSE] -> w387
            tunnel: w386 -> [w398 w479]
            tunnel: w385 -> [w404 w478]
            tunnel: [w406 _] -> w380
            tunnel: [w400 w477] -> w383
            tunnel: [w391 w479] -> w382
            frame No Error {
              n143 = call "Bytes at port more than X.vi"("X"=u32 100, "error IO"=w432, "port in"=w404) -> ("port out"=w431:refnum<visa-resource-name>, "Bytes at port > X"=w450:bool, "error out"=w430:errorcluster)  [unwired: 1 in, 3 out]
              n144 = call "Flush if true.vi"("error in"=w430, "Bytes at port > X"=w450, "port in"=w431) -> ("error out"=w449:errorcluster, "port out"=w448:refnum<visa-resource-name>)  [unwired: 1 in, 6 out]
              n145 = call "Bytes at port more eq 0 or less X.vi"("X"=u32 6, "serial ref  name"=w448, "error IO"=w449) -> ("Bytes at port <X or = 0?"=w410:bool, "serial out"=w444:refnum<visa-resource-name>, "Num. of Bytes at Port"=w446:u32, "error out"=w445:errorcluster)  [unwired: 2 in, 11 out]
              n146 = case shown="False" w410 {
                tunnel: w445 -> [w473 w475]
                tunnel: w446 -> [w472 _]
                tunnel: w444 -> [w471 w476]
                tunnel: [w470 w476] -> w441
                tunnel: [w469 _] -> w442
                tunnel: [w468 w475] -> w402
                tunnel: [w467 w474] -> w399
                tunnel: w398 -> [w467 w474]
                frame False {
                  n147 = VISA Read(VISA resource name=w471, byte count=w472, error in (no error)=w473) -> (VISA resource name out=w470:refnum<visa-resource-name>, read buffer=w469:string, error out=w468:errorcluster)  [unwired: 1 out]
                }
                frame True {
                }
              }
              n148 = Bundle("read buffer"=w442, "serial out"=w441, "error out"=w402, "occurrence"=w399) -> (w401:T7)  [unwired: 1 out]
              n149 = Unbundle(w401) -> ("read buffer"=w437:string, "serial out"=w436:refnum<visa-resource-name>, "error out"=w443:errorcluster, "occurrence"=w415:refnum<k4>)
              n150 = call "Match Axis NEW (SubVI).vi"("Axis ID"="^x", "input string"=w437, "Visa name in"=w436, "error in"=w443) -> ("Good\nto read!"=w428:bool, "out number"=w438:dbl, "out string"=w425:string, "Visa name out"=w424:refnum<visa-resource-name>, "error out"=w423:errorcluster)  [unwired: 3 in, 4 out]
              n151 = property on="RXd number" class="DigNum (strict)"() -> ("Value"=w408:u64)  [unwired: 2 in, 2 out]
              n152 = Bundle("out string"=w425, "Visa name out"=w424, "error out"=w423, "occurrence"=w415) -> (w422:T8)  [unwired: 1 in]
              n153 = case shown="True" w428 {
                tunnel: w438 -> [_ w462]
                tunnel: w422 -> [w461 w466]
                tunnel: [w461 w466] -> w421
                tunnel: [w460 w464] -> w409
                tunnel: w408 -> [w460 w465]
                frame False {
                }
                frame True {
                  n154 = Increment(x=w465) -> (x+1=w464:u64)
                  n155 = local write "Measurment Fl"(TRUE ("Measurment Fl")) -> ()
                  "Bx" <- w462
                }
              }
              n156 = property on="RXd number" class="DigNum (strict)"("Value"=w409) -> ()  [unwired: 2 in, 2 out]
              n157 = Unbundle(w421) -> ("out string"=w395:string, "Visa name out"=w394:refnum<visa-resource-name>, "error out"=w393:errorcluster, "occurrence"=w396:refnum<k4>)
              n158 = call "Match Axis NEW (SubVI).vi"("Axis ID"="^y", "input string"=w395, "Visa name in"=w394, "error in"=w393) -> ("Good\nto read!"=w427:bool, "out number"=w435:dbl, "out string"=w420:string, "Visa name out"=w419:refnum<visa-resource-name>, "error out"=w418:errorcluster)  [unwired: 1 in, 6 out]
              n159 = Bundle("out string"=w420, "Visa name out"=w419, "error out"=w418, "occurrence"=w396) -> (w417:T8)  [unwired: 1 in]
              n160 = case shown="True" w427 {
                tunnel: w435 -> [_ w458]
                tunnel: w417 -> [w457 w459]
                tunnel: [w457 w459] -> w416
                frame False {
                }
                frame True {
                  "By" <- w458
                }
              }
              n161 = Unbundle(w416) -> ("out string"=w390:string, "Visa name out"=w389:refnum<visa-resource-name>, "error out"=w388:errorcluster, "occurrence"=w392:refnum<k4>)
              n162 = call "Match Axis NEW (SubVI).vi"("Axis ID"="^z", "input string"=w390, "Visa name in"=w389, "error in"=w388) -> ("Good\nto read!"=w426:bool, "out number"=w397:dbl, "Visa name out"=w414:refnum<visa-resource-name>, "status"=w412:bool, "error out"=w413:errorcluster)  [unwired: 1 in, 6 out]
              n163 = Bundle("Visa name out"=w414, "error out"=w413, "status"=w412, "occurrence"=w392) -> (w411:T9)  [unwired: 1 out]
              n164 = case shown="True" w426 {
                tunnel: w397 -> [_ w455]
                tunnel: w411 -> [w454 w456]
                tunnel: [w454 w456] -> w407
                frame False {
                }
                frame True {
                  "Bz" <- w455
                }
              }
              n165 = local read "Стоп"() -> (w447:bool)
              n166 = Unbundle(w407) -> ("Visa name out"=w406:refnum<visa-resource-name>, "error out"=w400:errorcluster, "status"=w405:bool, "occurrence"=w391:refnum<k4>)
              n167 = Select(t=Magmeter."Stop" ("Beginning State"), s=w447, f=Magmeter."Read port" ("Beginning State")) -> (s? t:f=w451:T2)
              n168 = Not(x=w405) -> (.not. x?=w403:bool)
            }
            frame Error {
              n169 = VISA Close(VISA resource name=w478, error in (no error)=w484) -> (error out=w477:errorcluster)
              n170 = local read "Стоп"() -> (w483:bool)
              n171 = Select(t=Magmeter."Stop" ("Beginning State"), s=w483, f=Magmeter."Initialize" ("Beginning State")) -> (s? t:f=w480:T2)
            }
          }
          "Соединение" <- w387
        }
        frame "Write port" {
          n172 = call <vilib>:"Set Busy.vi"("error in (no error)"=w493) -> ("error out"=w494:errorcluster)  [unwired: 3 in, 7 out]
          n173 = call "Flush if true.vi"("error in"=w494, "Bytes at port > X"=FALSE, "port in"=w495) -> ("error out"=w500:errorcluster, "port out"=w499:refnum<visa-resource-name>)  [unwired: 1 in, 6 out]
          n174 = case shown="No Error" w500 {
            selector: w500 -> [w508 w513]
            tunnel: [w510 w512] -> w491
            tunnel: [w509 w513] -> w490
            tunnel: w499 -> [w507 w512]
            tunnel: w497 -> [w505 w511]
            tunnel: [w505 w511] -> w488
            frame No Error {
              # "Write bytes to port."
              n175 = VISA Write(VISA resource name=w507, write buffer="z", error in (no error)=w508) -> (VISA resource name out=w510:refnum<visa-resource-name>, error out=w509:errorcluster)  [unwired: 1 out]
            }
            frame Error {
            }
          }
          n176 = flat-sequence {
            tunnel: w491 -> [w504]
            tunnel: [w504] -> w487
            tunnel: w490 -> [w503]
            tunnel: [w503] -> w489
            tunnel: w488 -> [w502]
            tunnel: [w502] -> w486
            frame #0 {
              n177 = Wait (ms)(milliseconds to wait=u32 1500) -> ()  [unwired: 1 out]
            }
          }
          n178 = call <vilib>:"Unset Busy.vi"("error in (no error)"=w489) -> ("error out"=w492:errorcluster)  [unwired: 1 in, 9 out]
        }
      }
      n179 = Set Occurrence(w316) -> ()
      n180 = case shown="True" "Уст. ноль" {
        tunnel: w321 -> [w332 _]
        tunnel: [w332 Magmeter."Write port" ("Beginning State")] -> w320
        tunnel: [w331 w334] -> w318
        tunnel: w317 -> [w331 w334]
        tunnel: w315 -> [w330 w333]
        tunnel: [w330 w333] -> w314
        frame False {
        }
        frame True {
        }
      }
      n181 = property on="i" class="DigNum (strict)"(error in=w314, "Value"=w325) -> (error out=w324:errorcluster)  [unwired: 1 in, 1 out]
      n182 = Wait Until Next ms Multiple(millisecond multiple=u32 2) -> ()  [unwired: 1 out]
      n183 = call <vilib>:"General Error Handler.vi"("type of dialog (OK msg:1)"=u8 0 ("Disabled"), "error in (no error)"=w324) -> ("message"=→"Err msg":string, "error out"=w312:errorcluster)  [unwired: 12 out]
    }
    n184 = while {
      tunnel: w14 -> [w279]
      stop <- FALSE stop-if-true
      n185 = property on="Магнитные измерения" class="WFChart (strict)"() -> (error out=w248:errorcluster, "XScale.Maximum"=w253:dbl)  [unwired: 2 in, 1 out]
      n186 = Wait on Occurrence(1:FALSE ("ignore previous (T)"), 2:w279) -> ()  [unwired: 1 in, 1 out]
      n187 = property on="Магнитные измерения" class="WFChart (strict)"("Active Plot"=u32 0) -> (error out=w258:errorcluster)  [unwired: 2 in, 1 out]
      n188 = local read "Dx Sum"() -> (w255:u64)
      n189 = Greater Or Equal?(x=w255, y=w253) -> (x >= y?=w254:bool)
      n190 = case shown="True" w254 {
        tunnel: [w299 w303] -> w256
        tunnel: "Измерений\n \nна графике" -> [w298 w302]
        tunnel: w248 -> [w297 w301]
        tunnel: [w297 w300] -> w247
        frame False {
          n191 = Decrement "так как график стартует с 0"(x=w298) -> (x-1=w299:u16)
        }
        frame True {
          n192 = local read "Dz, мм"() -> (w304:u64)
          n193 = Add(x=w304, y=w302) -> (x+y=w303:u64)
          n194 = property on="Измерений\n \nна графике" class="DigNum (strict)"(error in=w301, "Value"=w303) -> (error out=w300:errorcluster)  [unwired: 1 in, 1 out]
        }
      }
      n195 = property on="Магнитные измерения" class="WFChart (strict)"(error in=w258, "Plot.Visible?"="Plot.Visible X") -> (error out=w281:errorcluster)  [unwired: 1 in, 1 out]
      n196 = property on="Магнитные измерения" class="WFChart (strict)"(error in=w281, "Active Plot"=u32 1) -> (error out=w277:errorcluster)  [unwired: 1 in, 1 out]
      n197 = property on="Магнитные измерения" class="WFChart (strict)"(error in=w247, "XScale.Maximum"=w256) -> (error out=w259:errorcluster)  [unwired: 1 in, 1 out]
      n198 = property on="Магнитные измерения" class="WFChart (strict)"(error in=w277, "Plot.Visible?"="Plot.Visible Y") -> (error out=w261:errorcluster)  [unwired: 1 in, 1 out]
      n199 = property on="Магнитные измерения" class="WFChart (strict)"(error in=w259, "XScale.Minimum"=0.0 ("X Scale.Range:Minimum")) -> (error out=w257:errorcluster)  [unwired: 1 in, 1 out]
      n200 = case shown="False" "Графики толще" {
        tunnel: [u8 0 ("Plot.Line Width") u8 3 ("Plot.Line Width")] -> w265
        frame False {
        }
        frame True {
        }
      }
      n201 = property on="Магнитные измерения" class="WFChart (strict)"(error in=w257, "Active Plot"=u32 0) -> (error out=w260:errorcluster)  [unwired: 1 in, 1 out]
      n202 = property on="Магнитные измерения" class="WFChart (strict)"(error in=w261, "Active Plot"=u32 2) -> (error out=w283:errorcluster)  [unwired: 1 in, 1 out]
      n203 = case shown="True" "Маркеры" {
        tunnel: [w306 w308] -> w251
        tunnel: w265 -> [w306 w308]
        tunnel: [u8 0 ("Plot.Line Width") u8 5 ("Plot.Line Width")] -> w263
        frame False {
        }
        frame True {
        }
      }
      n204 = property on="Магнитные измерения" class="WFChart (strict)"(error in=w260, "Plot.Line Width"=w251) -> (error out=w269:errorcluster)  [unwired: 1 in, 1 out]
      n205 = property on="Магнитные измерения" class="WFChart (strict)"(error in=w283, "Plot.Visible?"="Plot.Visible Z") -> (error out=w246:errorcluster)  [unwired: 1 in, 1 out]
      n206 = property on="Магнитные измерения" class="WFChart (strict)"(error in=w269, "Plot.Point Style"=w263) -> (error out=w270:errorcluster)  [unwired: 1 in, 1 out]
      n207 = property on="Магнитные измерения" class="WFChart (strict)"(error in=w270, "Active Plot"=u32 1) -> (error out=w275:errorcluster)  [unwired: 1 in, 1 out]
      n208 = property on="Магнитные измерения" class="WFChart (strict)"(error in=w275, "Plot.Line Width"=w251) -> (error out=w267:errorcluster)  [unwired: 1 in, 1 out]
      n209 = property on="Table num index" class="DigNum (strict)"(error in=w246) -> (error out=w239:errorcluster, "Value"=w244:u32)  [unwired: 1 in, 1 out]
      n210 = Equal To 0?(x=w244) -> (x = 0?=w243:bool)
      n211 = case shown="True" w243 {
        tunnel: [u32 0 ("Table num index") u32 2 ("Table num index")] -> w242
        tunnel: w239 -> [w293 w295]
        tunnel: [w293 w295] -> w238
        frame False {
        }
        frame True {
        }
      }
      n212 = property on="Магнитные измерения" class="WFChart (strict)"(error in=w267, "Plot.Point Style"=w263) -> (error out=w268:errorcluster)  [unwired: 1 in, 1 out]
      n213 = property on="Удалить измерение" class="Bool (strict)"(error in=w238, "Disabled"=w242) -> (error out=w235:errorcluster)  [unwired: 1 in, 1 out]
      n214 = property on="Магнитные измерения" class="WFChart (strict)"(error in=w268, "Active Plot"=u32 2) -> (error out=w272:errorcluster)  [unwired: 1 in, 1 out]
      n215 = property on="Магнитные измерения" class="WFChart (strict)"(error in=w272, "Plot.Line Width"=w251) -> (error out=w266:errorcluster)  [unwired: 1 in, 1 out]
      n216 = case shown="True" "Автосохранение" {
        tunnel: [u8 2 ("Plot.Line Width") u8 0 ("Plot.Line Width")] -> w241
        tunnel: w235 -> [w289 w291]
        tunnel: [w289 w291] -> w240
        frame False {
        }
        frame True {
        }
      }
      n217 = property on="Магнитные измерения" class="WFChart (strict)"(error in=w266, "Plot.Point Style"=w263) -> (error out=w237:errorcluster)  [unwired: 1 in, 1 out]
      n218 = property on="Интервал \n\n[сек.]" class="DigNum (strict)"(error in=w240, "Disabled"=w241) -> (error out=w234:errorcluster)  [unwired: 1 in, 1 out]
      n219 = Wait Until Next ms Multiple(millisecond multiple=u32 10) -> ()  [unwired: 1 out]
      n220 = Merge Errors(w237, w234) -> (w249:errorcluster)
      n221 = call <vilib>:"Simple Error Handler.vi"("type of dialog (OK msg:1)"=u32 0 ("Table num index"), "error in (no error)"=w249) -> ()  [unwired: 8 out]
    }
  }
